vi "Find New DVR Node.vi"(8 "error in (no error)":errorcluster, 11 "VI Refnum":refnum<vi>) -> (0 "error out":errorcluster, 2 "Found?":bool, 3 "New DVR Node":refnum<vi>)   [LabVIEW 2018, in "LVClassByRef.lvlib"]
uses:
  <resource>/Framework/Providers/LVClassByRef/LVClassByRef.lvlib
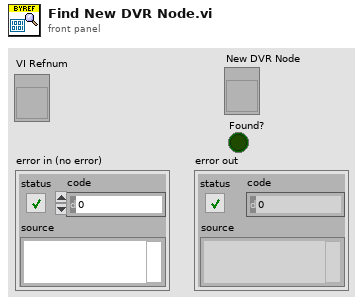
[diagram p1: front panel]
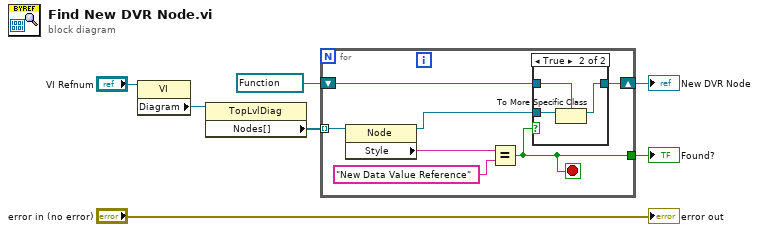
[diagram p0: block diagram]
diagram:
  n1 = property class="VI"(reference="VI Refnum") -> ("Diagram"=w6:refnum<vi>)  [unwired: 1 in, 2 out]
  n2 = property class="TopLvlDiag"(reference=w6) -> ("Nodes[]"=w5:refnum<vi>[])  [unwired: 1 in, 2 out]
  n3 = for {
    tunnel: w5 -> [w14] mode=indexing
    shift-right: [w8] -> w2
    shift-left: refnum<vi> refnum ("f") -> [w9]
    tunnel: [w11] -> w3
    stop <- w11 stop-if-true
    n4 = property class="Node"(reference=w14) -> (reference out=w10:refnum<vi>, "Style"=w12:string)  [unwired: 1 in, 1 out]
    n5 = Equal?(x=w12, y="New Data Value Reference") -> (x = y?=w11:bool)
    n6 = case shown="True" w11 {
      tunnel: w10 -> [_ w18]
      tunnel: w9 -> [w15 w17]
      tunnel: [w15 w16] -> w8
      frame False {
      }
      frame True {
        n7 = To More Specific Class(target class=w17, reference=w18) -> (specific class reference=w16:refnum<vi>)  [unwired: 1 in, 1 out]
      }
    }
  }
  "Found?" <- w3
  "New DVR Node" <- w2
  "error out" <- "error in (no error)"
